vi "GraphsUpdateMean.vi"(9 "runs":i32=10, 10 "All new data in":dbl[][](array[numeric]), 11 "GraphChart in":refnum<vi>) -> ()   [LabVIEW 2017]
uses:
  <vilib>/Analysis/baseanly.llb/Mean (DBL).vi
  controls/GlobalExp.vi
  <vilib>/Analysis/NI_AALBase.lvlib
  Global.lvlib
panel:
  out "Waveform Graph":dbl[][](graph)
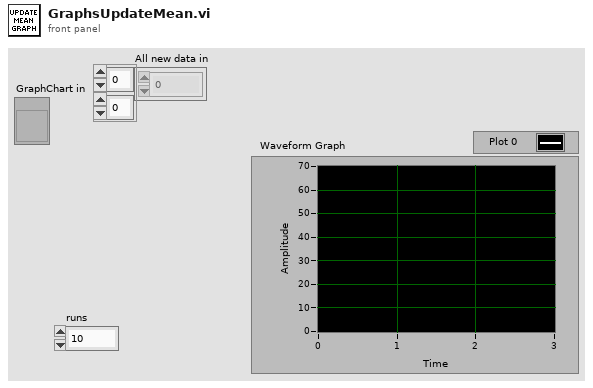
[diagram p1: front panel]
types:
  T1 = typedef "MasterExpControl.ctl" = cluster{"Main Steps":dbl, "Main Runs":dbl, "ExpStatus":enum16{"Innit", "Stop", "Idle", "MainRunning", "AuxRunning"}, "Main Current Step":dbl, "ExpNum":dbl, "NewData":bool, "date":string, "command":string, "Stop":bool, "Pause":bool, "Mathematica":string, "Main/Meta":bool, "UpdateMath":bool, "Camera":bool, "MetaExpOver":bool}
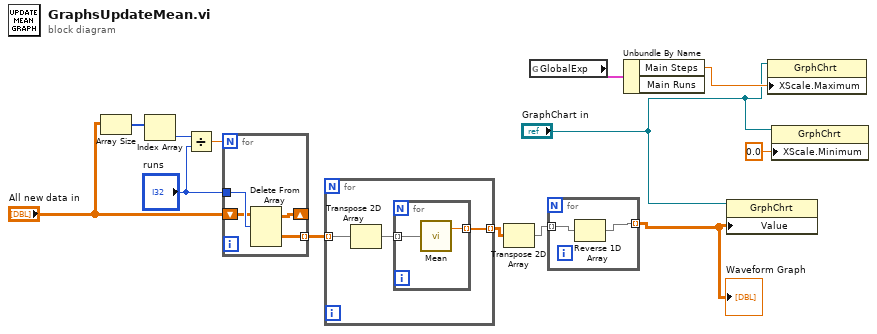
[diagram p0: block diagram]
diagram:
  n1 = Array Size(array="All new data in") -> (size(s)=w13:i32[])
  n2 = Index Array(array=w13) -> (element=w12:i32)  [unwired: 1 in]
  n3 = Divide(x=w12, y="runs") -> (x/y=w11:dbl)
  n4 = for {
    N: w11 -> [_]
    shift-right: [w14] -> _
    shift-left: "All new data in" -> [w16]
    tunnel: "runs" -> [w17]
    tunnel: [w15] -> w8 mode=indexing
    n5 = Delete From Array(array=w16, length=w17) -> (deleted portion=w15:dbl[][], array with subset deleted=w14:dbl[][])  [unwired: 2 in]
  }
  n6 = for {
    tunnel: w8 -> [w19] mode=indexing
    tunnel: [w20] -> w3 mode=indexing
    n7 = Transpose 2D Array(2D array=w19) -> (transposed array=w18:dbl[][])
    n8 = for {
      tunnel: w18 -> [w22] mode=indexing
      tunnel: [w21] -> w20 mode=indexing
      n9 = call-poly <vilib>:"Mean.vi"("X"=w22) -> ("mean"=w21:dbl)  [unwired: 1 out]
    }
  }
  n10 = Transpose 2D Array(2D array=w3) -> (transposed array=w2:dbl[][])
  n11 = global read "GlobalExp.vi" "GlobalExp"() -> (w7:T1)
  n12 = for {
    tunnel: w2 -> [w24] mode=indexing
    tunnel: [w23] -> w1 mode=indexing
    n13 = Reverse 1D Array(array=w24) -> (reversed array=w23:dbl[])
  }
  "Waveform Graph" <- w1
  n14 = Unbundle By Name(w7) -> ("Main Steps"=w6:dbl)  [unwired: 1 out]
  n15 = property class="GrphChrt"(reference="GraphChart in", "Value"=w1) -> ()  [unwired: 1 in, 2 out]
  n16 = property class="GrphChrt"(reference="GraphChart in", "XScale.Maximum"=w6) -> ()  [unwired: 1 in, 2 out]
  n17 = property class="GrphChrt"(reference="GraphChart in", "XScale.Minimum"=0.0 ("X Scale.Range:Minimum")) -> ()  [unwired: 1 in, 2 out]
